vi "FBLooseVI.vi"(11 "x":dbl(slide)=10.0 scale=0.0..10.0) -> (3 "2x^2":dbl=200.0)   [LabVIEW 2023]
doc: "Input = x\nOutput = 2x^2"
panel:
  out "x":dbl=10.0
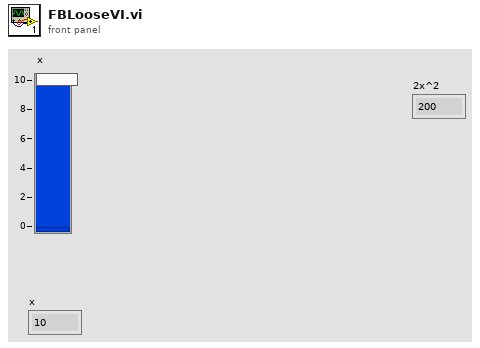
[diagram p1: front panel]
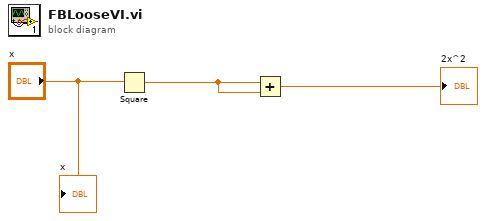
[diagram p0: block diagram]
diagram:
  n1 = Square(x="x") -> (x^2=w3:dbl)
  n2 = Add(x=w3, y=w3) -> (x+y=→"2x^2":dbl)
  "x" <- "x"
